vi "Prechirper command process.vi"(10 "Data to Set":dbl, 11 "Pre-chirper commands":T1) -> (3 "Comand String":string)   [LabVIEW 2017]
uses:
  Prechirper commands.ctl
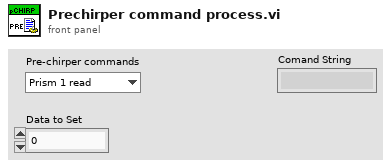
[diagram p1: front panel]
types:
  T1 = typedef "Prechirper commands.ctl" = enum16{"Prism 1 read", "Prism 1 set", "Prism 2 read", "Prism 2 set", "Wavelength read", "Wavelength Femto set", "Wavelength Femto and Laser set", "GVD curve number read", "GVD curve number set"}
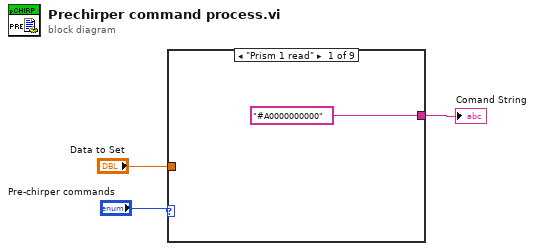
[diagram p0: block diagram]
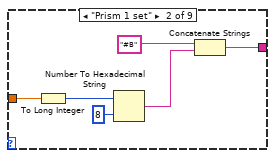
[diagram p2: hidden frame]
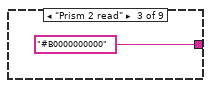
[diagram p3: hidden frame]
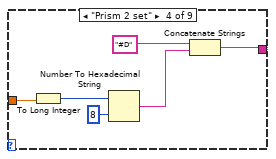
[diagram p4: hidden frame]
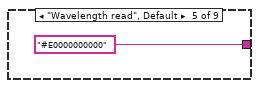
[diagram p5: hidden frame]
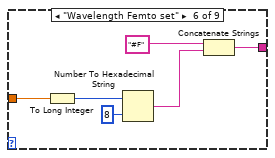
[diagram p6: hidden frame]
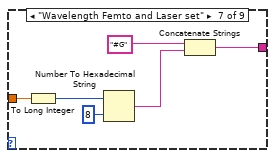
[diagram p7: hidden frame]
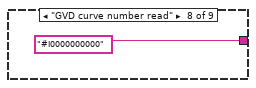
[diagram p8: hidden frame]
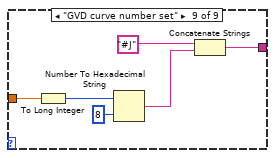
[diagram p9: hidden frame]
diagram:
  n1 = case shown="\"Prism 1 read\"" "Pre-chirper commands" {
    tunnel: "Data to Set" -> [_ w10 _ w13 _ w20 w26 _ w33]
    tunnel: ["#A0000000000" w5 "#B0000000000" w12 "#E0000000000" w19 w25 "#I0000000000" w32] -> w1
    frame "Prism 1 read" {
    }
    frame "Prism 1 set" {
      n2 = To Long Integer(number=w10) -> (32bit integer=w9:i32)
      n3 = Number To Hexadecimal String(1:i16 8 ("width (-)"), 2:w9) -> (0:w6:string)
      n4 = Concatenate Strings("#B", w6) -> (w5:string)
    }
    frame "Prism 2 read" {
    }
    frame "Prism 2 set" {
      n5 = To Long Integer(number=w13) -> (32bit integer=w17:i32)
      n6 = Number To Hexadecimal String(1:i16 8 ("width (-)"), 2:w17) -> (0:w14:string)
      n7 = Concatenate Strings("#D", w14) -> (w12:string)
    }
    frame "Wavelength read", Default {
    }
    frame "Wavelength Femto set" {
      n8 = To Long Integer(number=w20) -> (32bit integer=w24:i32)
      n9 = Number To Hexadecimal String(1:i16 8 ("width (-)"), 2:w24) -> (0:w21:string)
      n10 = Concatenate Strings("#F", w21) -> (w19:string)
    }
    frame "Wavelength Femto and Laser set" {
      n11 = To Long Integer(number=w26) -> (32bit integer=w30:i32)
      n12 = Number To Hexadecimal String(1:i16 8 ("width (-)"), 2:w30) -> (0:w27:string)
      n13 = Concatenate Strings("#G", w27) -> (w25:string)
    }
    frame "GVD curve number read" {
    }
    frame "GVD curve number set" {
      n14 = To Long Integer(number=w33) -> (32bit integer=w37:i32)
      n15 = Number To Hexadecimal String(1:i16 8 ("width (-)"), 2:w37) -> (0:w34:string)
      n16 = Concatenate Strings("#J", w34) -> (w32:string)
    }
  }
  "Comand String" <- w1
